vi "FPGA - Select Bitfile (Local).vi"(8 "error in (no error)":errorcluster, 11 "Node Ptr":u64 format="%.0x") -> (0 "error out":errorcluster)   [LabVIEW 2019, in "SEECD System Explorer.lvlib"]
uses:
  Type Defs/FPGA Target.ctl
  Shared/Type Defs/Host - FPGAScanInterfaceMode.ctl
  SEECD System Explorer.lvlib
  <vilib>/NI VeriStand/Custom Device Tools/Custom Device Utility Library/Custom Device Utility Library.lvlib
  Shared/SEECD Shared.lvlib
  <vilib>/NI VeriStand/Custom Device API/Custom Device API.lvlib
panel:
  in  "Tag":string
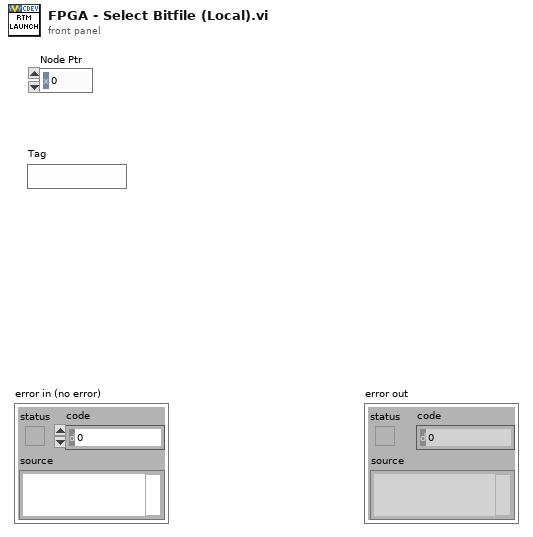
[diagram p1: front panel]
types:
  T1 = typedef "SEECD Shared.lvlib/Host - FPGAScanInterfaceMode.ctl" = enum16{"Use Current", "FPGA", "Scan Mode"}
  T2 = typedef "SEECD System Explorer.lvlib/FPGA Target.ctl" = enum16{"Local", "EtherCAT"}
  T3 = typedef "Custom Device API.lvlib/Custom Device Item Ref.ctl" = u64
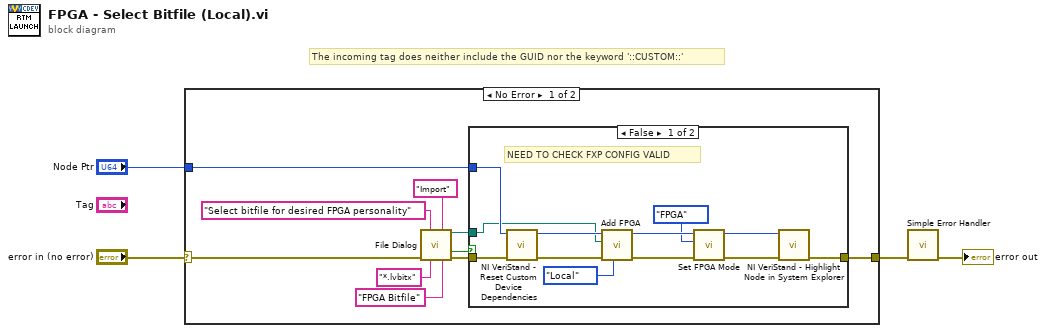
[diagram p0: block diagram]
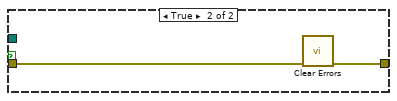
[diagram p2: hidden frame]
diagram:
  # "The incoming tag does neither include the GUID nor the keyword '::CUSTOM::'"
  n1 = case shown="No Error" "error in (no error)" {
    selector: "error in (no error)" -> [w6 w29]
    tunnel: "Node Ptr" -> [w5 _]
    tunnel: [w7 w29] -> w2
    frame No Error {
      n2 = call "File Dialog"("prompt"="Select bitfile for desired FPGA personality", "button label"="Import", "error in"=w6, "pattern (all files)"="*.lvbitx", "pattern label"="FPGA Bitfile") -> ("selected path"=w14:path, "cancelled"=w12:bool, "error out"=w13:errorcluster)  [unwired: 7 in, 1 out]
      n3 = case shown="False" w12 {
        tunnel: w13 -> [w19 w28]
        tunnel: w14 -> [w15 _]
        tunnel: [w25 w27] -> w7
        tunnel: w5 -> [w18 _]
        frame False {
          # "NEED TO CHECK FXP CONFIG VALID"
          n4 = call <vilib>:"NI VeriStand - Reset Custom Device Dependencies.vi"("error in (no error)"=w19, "Device Ref in"=w18) -> ("error out"=w16:errorcluster, "Device Ref out"=w17:T3)  [unwired: 8 in]
          n5 = call "Add FPGA.vi"("FPGA Target"=FPGA_Target."Local", "error in (no error)"=w16, "Bitfile Path"=w15, "Item Ref in"=w17) -> ("error out"=w23:errorcluster, "Item Ref out"=w24:T3)  [unwired: 6 in]
          n6 = call "Set FPGA Mode.vi"("error in (no error)"=w23, "FPGAScanInterfaceMode"=Host_-_FPGAScanInterfaceMode."FPGA", "Item Ref in"=w24) -> ("error out"=w20:errorcluster, "Item Ref out"=w21:T3)  [unwired: 7 in]
          n7 = call <vilib>:"NI VeriStand - Highlight Node in System Explorer.vi"("error in (no error)"=w20, "Item Ref in"=w21) -> ("error out"=w25:errorcluster)  [unwired: 8 in, 1 out]
        }
        frame True {
          n8 = call <vilib>:"Clear Errors.vi"("error in (no error)"=w28) -> ("error out"=w27:errorcluster)  [unwired: 1 in, 5 out]
        }
      }
    }
    frame Error {
    }
  }
  n9 = call <vilib>:"Simple Error Handler.vi"("error in (no error)"=w2) -> ("error out"=→"error out":errorcluster)  [unwired: 4 in, 4 out]
